vi "SV TDMS Write Scalar (N Ch).vi"(0 "tdms file":refnum<k34>, 1 "write channel properties (T)":bool=TRUE, 5 "group name in (Feature)":string="Feature", 7 "channel names in":string[](array[string]), 9 "values in":dbl[](array[numeric]), 11 "error in":errorcluster, 12 "scalar function info in":T1={"scalar function type"=10, "scalar function subtype"=19, " x-dimension"=0} {"scalar function type" items=["Speed"=3, "Ratio"=6, "Count"=7, "-"=9, "Level"=10, "-"=19, "None"=98]; "scalar function subtype" items=["Value"=19, "DC"=11, "AC"=12, "RMS^2"=13, "RMS"=14, "Peak"=15, "Peak to peak"=16, "-"=20, "Phase"=33, "-"=90, "None"=98, "Unknown"=99]; "x-dimension" items=["Time (s)"=0, "Frequency-CB (Hz)"=1, "Frequency-CPB (Hz)"=1248, "Frequency-Arbitrary (Hz)"=2357, "Quefrency (s)"=2, "Revolutions (rev)"=3, "Order"=4, "Speed (RPM)"=11, "Speed (rad/s)"=21, "Critical Band"=31, "Critical Band Rate (Bark)"=32, "None"=98, "Index"=65535]}, 13 "Y-unit label (\"\")":string[](array[string])) -> (4 "tdms file out":refnum<k34>, 6 "group name out":string, 8 "channel names out":string[](array[string]), 15 "error out":errorcluster)   [LabVIEW 2017]
doc: "Writes data to the specified .tdms file in a format specific to the polymorphic instance. Wire data to the <B>scaled signal [EU]</B> input to determine the polymorphic instance to use or manually select the instance."
uses:
  <vilib>/addons/_NISVFA/_Shared subVIs/Controls/NI Scalar Function Info.ctl
  <vilib>/addons/_NISVFA/_Shared subVIs/Controls/svc_X-Axis Units.ctl
  <vilib>/addons/_NISVFA/_Shared subVIs/Controls/LV Datatypes.ctl
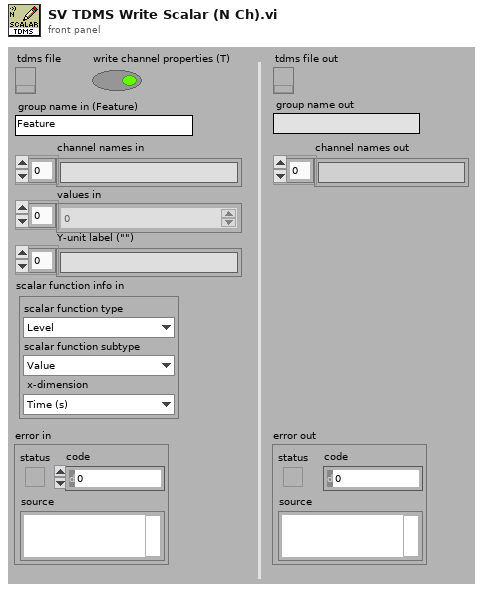
[diagram p1: front panel]
types:
  T1 = typedef "NI Scalar Function Info.ctl" = cluster{"scalar function type":u16, "scalar function subtype":u16, " x-dimension":T2}
  T2 = typedef "svc_X-Axis Units.ctl" = u16
  T3 = typedef "LV Datatypes.ctl" = i32
  T4 = typedef "svc_Unit Info.ctl" = cluster{"X-axis label":string, "X-unit string":string, "Y-axis label":string, "Y-unit string":string}
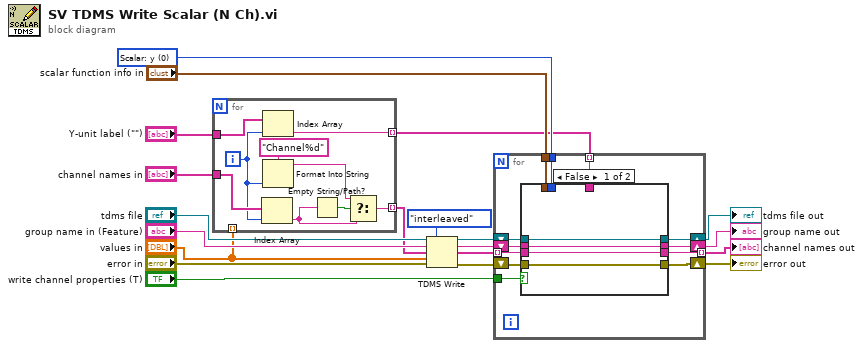
[diagram p0: block diagram]
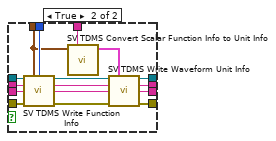
[diagram p2: hidden frame]
diagram:
  w15 = T3 0 items=["String: abc"=-2, "Boolean: True or False"=-1, "Scalar: y"=0, "Array: Y"=1, "Waveform: t0, dt, Y, variant"=2, "Cluster: x0, dx, Y"=3, "Cluster: X, Y"=4, "Waterfall"=5, "Colormap"=6] ("LabVIEW datatype")
  n1 = for {
    tunnel: "Y-unit label (\"\")" -> [w29]
    tunnel: "channel names in" -> [w23]
    tunnel: [w25] -> w8 mode=indexing
    tunnel: [w24] -> w3 mode=indexing
    tunnel: "values in" -> [_] mode=indexing
    i -> [w22]
    n2 = Index Array(array=w23, index=w22) -> (element=w21:string)
    n3 = Index Array(array=w29, index=w22) -> (element=w24:string)
    n4 = Format Into String(format string="Channel%d", w22) -> (resulting string=w28:string)  [unwired: 2 in, 1 out]
    n5 = Empty String/Path?(string/path=w21) -> (empty?=w26:bool)
    n6 = Select(t=w28, s=w26, f=w21) -> (s? t:f=w25:string)
  }
  n7 = TDMS Write(0:"tdms file", 1:enum16{"decimated", "interleaved"}."interleaved" ("data layout (0:decimated)"), 5:"group name in (Feature)", 7:w8, 9:"values in", 11:"error in") -> (4:w7:refnum<k34>, 6:w6:string, 8:w5:string[], 15:w4:errorcluster)
  n8 = for {
    tunnel: w15 -> [w41]
    tunnel: "write channel properties (T)" -> [w40]
    tunnel: [w37] -> w11 mode=indexing
    tunnel: "scalar function info in" -> [w35]
    tunnel: w5 -> [w32] mode=indexing
    tunnel: w3 -> [w30] mode=indexing
    shift-right: [w38] -> w12
    shift-left: w7 -> [w34]
    shift-right: [w39] -> w13
    shift-left: w6 -> [w33]
    shift-right: [w36] -> w10
    shift-left: w4 -> [w31]
    n9 = case shown="False" w40 {
      tunnel: w34 -> [w45 w57]
      tunnel: [w45 w56] -> w38
      tunnel: w33 -> [w44 w55]
      tunnel: w32 -> [w43 w54]
      tunnel: [w44 w53] -> w39
      tunnel: [w43 w52] -> w37
      tunnel: [w42 w51] -> w36
      tunnel: w31 -> [w42 w50]
      tunnel: w35 -> [_ w48]
      tunnel: w41 -> [_ w49]
      tunnel: w30 -> [_ w46]
      frame False {
      }
      frame True {
        n10 = call <vilib>:"SV TDMS Write Function Info.vi"("tdms file in"=w57, "function info"=w48, "LabVIEW datatype"=w49, "group name"=w55, "channel name"=w54, "error in (no error)"=w50) -> ("tdms file out"=w58:refnum<k34>, "group name out"=w59:string, "channel name out"=w60:string, "error out"=w61:errorcluster)  [unwired: 6 in]
        n11 = call <vilib>:"SV TDMS Convert Scalar Function Info to Unit Info.vi"("Y-unit string override"=w46, "scalar info in"=w48) -> ("unit info"=w47:T4)  [unwired: 9 in]
        n12 = call <vilib>:"SV TDMS Write Waveform Unit Info.vi"("tdms file"=w58, "unit info"=w47, "group name"=w59, "channel name"=w60, "error in (no error)"=w61) -> ("tdms file out"=w56:refnum<k34>, "group name out"=w53:string, "channel name out"=w52:string, "error out"=w51:errorcluster)  [unwired: 7 in]
      }
    }
  }
  "tdms file out" <- w12
  "error out" <- w10
  "channel names out" <- w11
  "group name out" <- w13
